vi "TSM DAQmx N Pins To M Tasks.vi"(0 "TSM context":T3, 5 "Pins":tag[](array[tag]), 7 "Site Numbers":i32[](array[numeric]), 11 "error in":errorcluster) -> (4 "DAQ TSM Out":T1, 15 "error out":errorcluster)   [LabVIEW 2020]
doc: "Populates the TSM SSC DAQmx cluster for the specified pin(s) and pin group(s)."
uses:
  <vilib>/NI_TestStand_SemiconductorModule/NI_TestStand_Semiconductor_Module.lvlibp/PinMap/General/SemiconductorModuleContext.ctl
  TSM DAQmx Multi-Task.ctl
  <vilib>/NI_TestStand_SemiconductorModule/NI_TestStand_Semiconductor_Module.lvlibp/PinMap/PinQueryContext/MultiplePinMultipleSessionQueryContext/MultiplePinMultipleSessionQueryContext.lvclass
  C:/Program Files/National Instruments/LabVIEW 2020/vi.lib/NI_TestStand_SemiconductorModule/NI_TestStand_Semiconductor_Module.lvlibp/PinMap/PinQueryContext/PinQueryContext.lvclass
  SSC DAQmx.ctl
  <vilib>/NI_TestStand_SemiconductorModule/NI_TestStand_Semiconductor_Module.lvlibp/PinMap/DAQmx/PinsToNIDAQmxTasks.vi
  <vilib>/NI_TestStand_SemiconductorModule/NI_TestStand_Semiconductor_Module.lvlibp
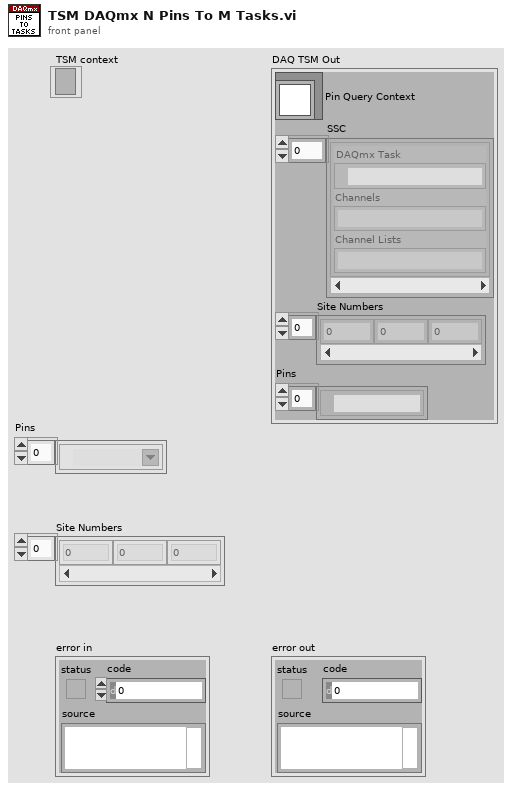
[diagram p1: front panel]
types:
  T1 = typedef "TSM DAQmx Multi-Task.ctl" = cluster{"Pin Query Context":refnum<class "MultiplePinMultipleSessionQueryContext.lvclass">, "SSC":T2[], "Site Numbers":i32[], "Pins":tag[]}
  T2 = typedef "SSC DAQmx.ctl" = cluster{"DAQmx Task ":refnum<k21>, "Channels":string, "Channel Lists":string}
  T3 = typedef "NI_TestStand_Semiconductor_Module.lvlibp/SemiconductorModuleContext.ctl" = refnum<k7>
  T4 = cluster{"DAQmx Task":refnum<k21>, "Channel List":string, "spreadsheet string":string}[]
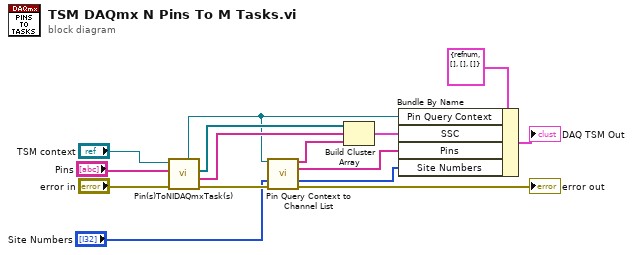
[diagram p0: block diagram]
diagram:
  n1 = call-poly <vilib>:"Pin(s)ToNIDAQmxTask(s).vi"("error in (no error)"="error in", "Pins"="Pins", "Semiconductor Module Context"="TSM context") -> ("error out"=w13:errorcluster, "Channel Lists"=w8:string[], "DAQmx Tasks"=w9:refnum<k21>[], "Pin Query Context"=w7:refnum<class "MultiplePinMultipleSessionQueryContext.lvclass">)  [unwired: 4 in, 1 out]
  n2 = call "Pin Query Context to Channel List.vi"("Pin Query Context"=w7, "Site Numbers In"="Site Numbers", "error in"=w13) -> ("Per-Session Channel List"=w6:string[], "Pins"=w1:tag[], "Site Numbers Out"=w2:i32[], "error out"=→"error out":errorcluster)  [unwired: 9 in]
  n3 = Build Cluster Array(w9, w8, w6) -> (w5:T4)
  n4 = Bundle By Name(cluster=T1 {"Pin Query Context"=refnum, "SSC"=[], "Site Numbers"=[], "Pins"=[]} ("DAQmx - Multiple Sessions Info"), "Pin Query Context"=w7, "SSC"=w5, "Pins"=w1, "Site Numbers"=w2) -> (→"DAQ TSM Out":T1)
